vi "Create.vi"(8 "error in (no error)":errorcluster, 9 "Current Log":refnum<notifier>, 10 "Log Folder":path, 11 "LogManager":refnum<class "MessageQ.lvclass">) -> (0 "error out":errorcluster, 3 "LogHTTPController out":refnum<class "LogHTTPController.lvclass">)   [LabVIEW 2020, in "VolatusData.lvlib" / "LogHTTPController.lvclass"]
uses:
  LogHTTPController.lvclass
  LogHTTPController.lvclass/LogHTTPController.ctl
  Volatus/MessageQ/MessageQ.lvclass
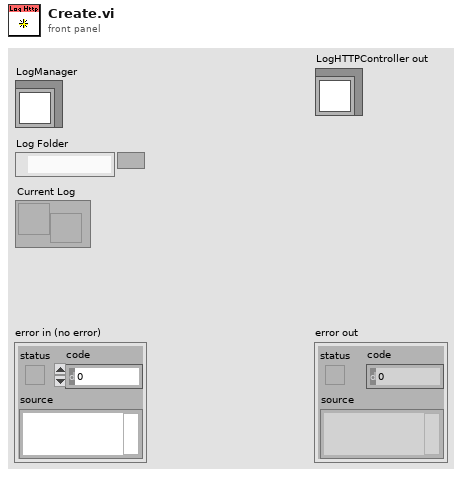
[diagram p1: front panel]
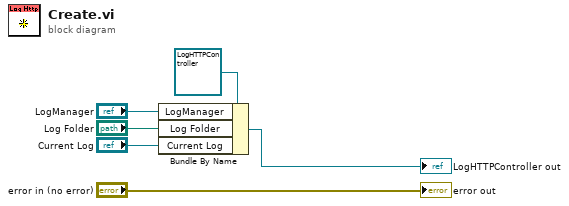
[diagram p0: block diagram]
diagram:
  n1 = Bundle By Name(cluster=refnum<class "LogHTTPController.lvclass"> refnum ("LogHTTPController in"), "LogManager"="LogManager", "Log Folder"="Log Folder", "Current Log"="Current Log") -> (→"LogHTTPController out":refnum<class "LogHTTPController.lvclass">)
  "error out" <- "error in (no error)"
